vi "digital time using leds.vi"() -> ()   [LabVIEW 2018]
panel:
  out "?":bool
  out "?":bool
  out "?":bool
  out "?":bool
  out "?":bool
  out "?":bool
  out "?":bool
  out "?":bool
  out "?":bool
  out "?":bool
  out "?":bool
  out "?":bool
  out "?":bool
  out "?":bool
  out "?":bool
  out "?":bool
  out "?":bool
  out "?":bool
  out "?":bool
  out "?":bool
  out "?":bool
  out "?":bool
  out "?":bool
  out "?":bool
  out "?":bool
  out "?":bool
  out "?":bool
  out "?":bool
  in  "stop":bool
  out "?":bool
  out "?":bool
  out "?":bool
  out "?":bool
  out "?":bool
  out "?":bool
  out "?":bool
  out "?":bool
  out "?":bool
  out "?":bool
  out "?":bool
  out "?":bool
  out "?":bool
  out "?":bool
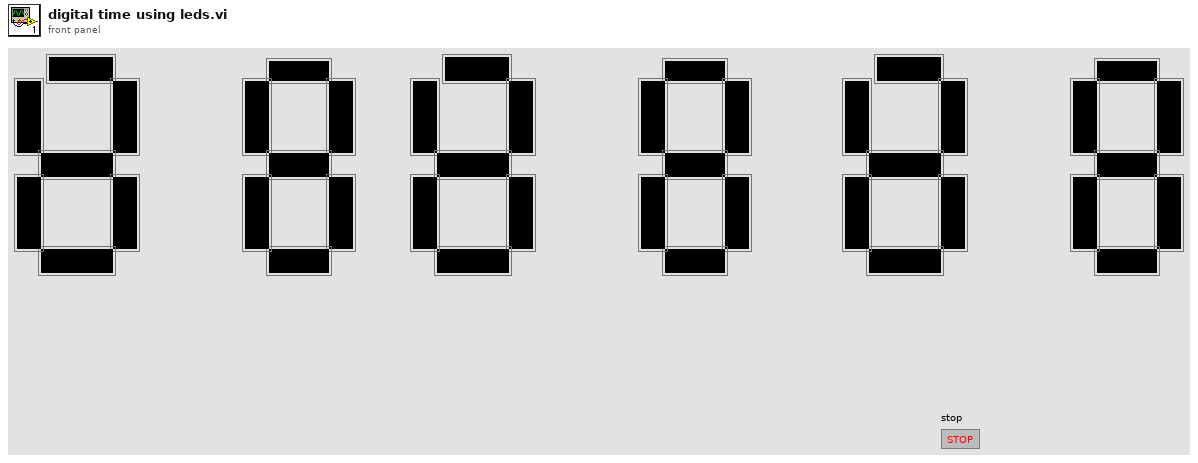
[diagram p1: front panel]
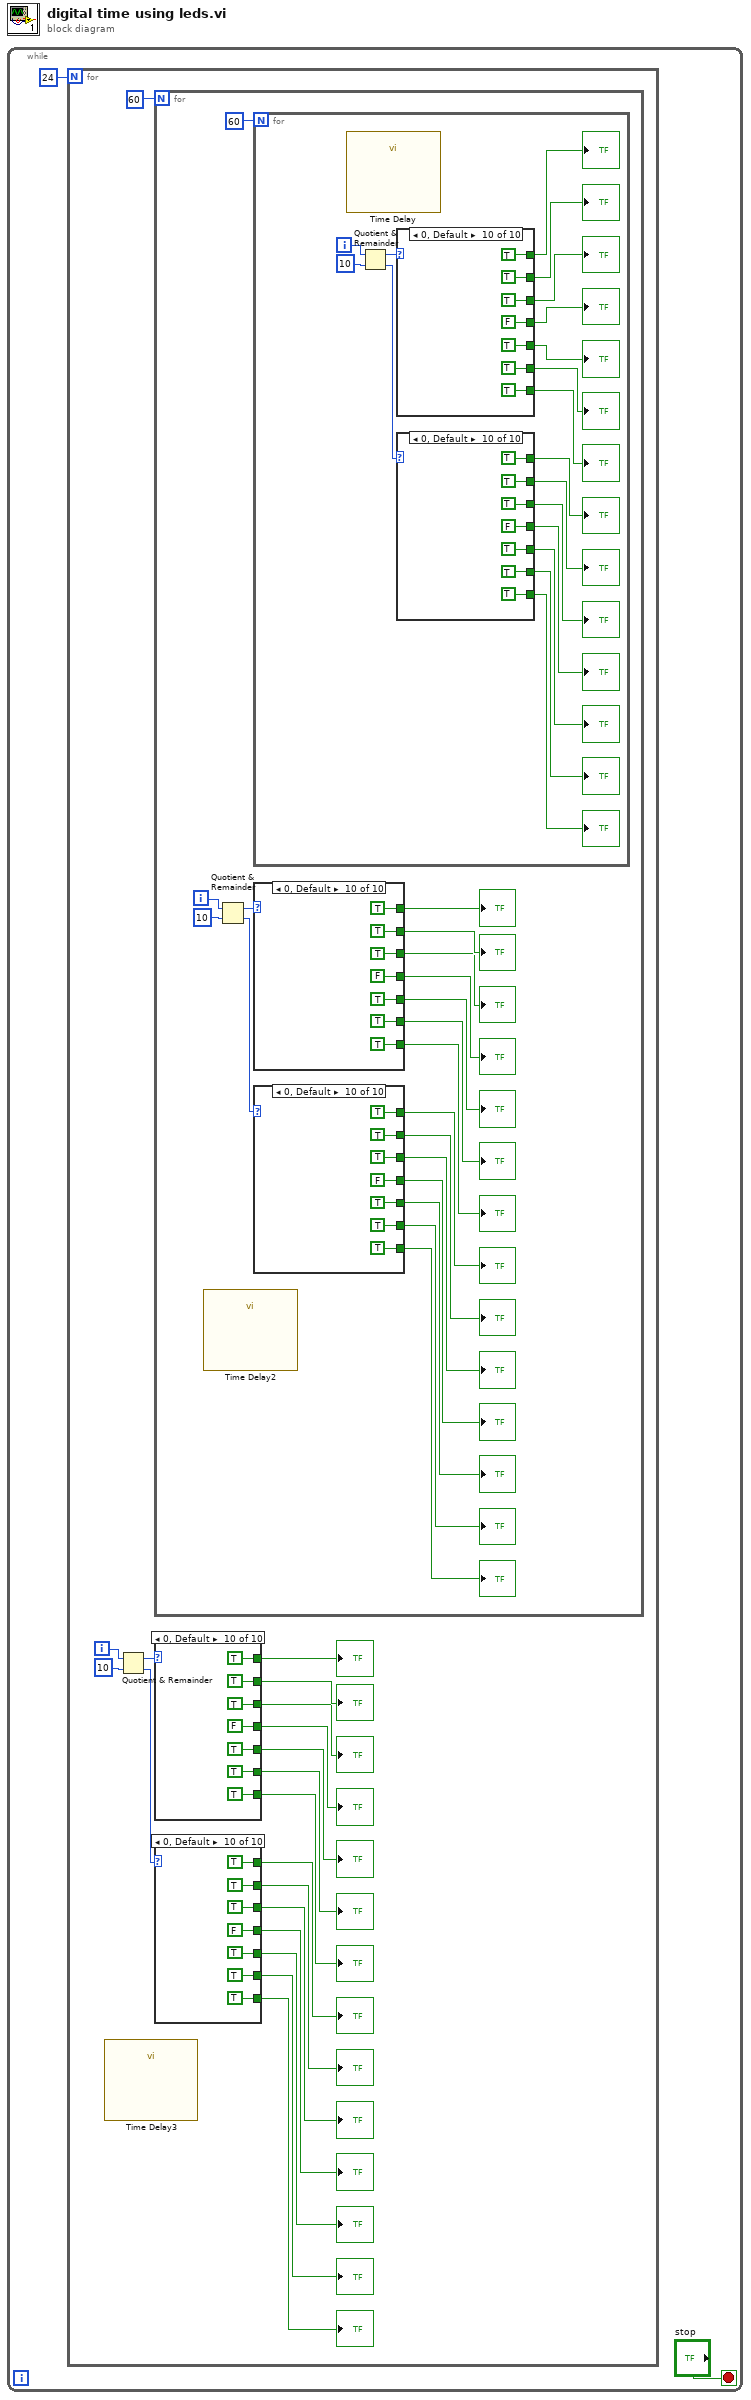
[diagram p0: block diagram]
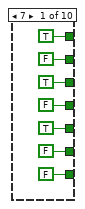
[diagram p2: hidden frame]
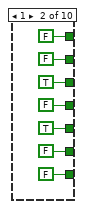
[diagram p3: hidden frame]
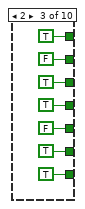
[diagram p4: hidden frame]
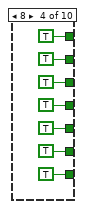
[diagram p5: hidden frame]
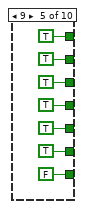
[diagram p6: hidden frame]
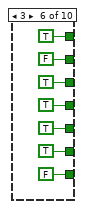
[diagram p7: hidden frame]
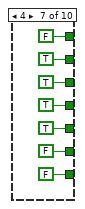
[diagram p8: hidden frame]
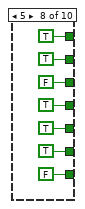
[diagram p9: hidden frame]
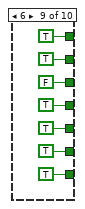
[diagram p10: hidden frame]
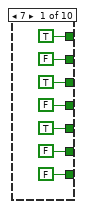
[diagram p11: hidden frame]
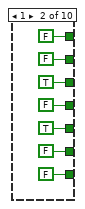
[diagram p12: hidden frame]
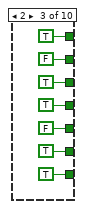
[diagram p13: hidden frame]
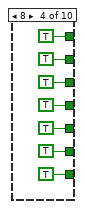
[diagram p14: hidden frame]
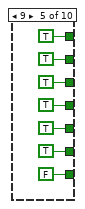
[diagram p15: hidden frame]
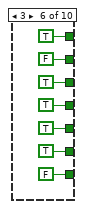
[diagram p16: hidden frame]
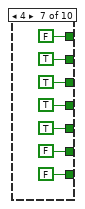
[diagram p17: hidden frame]
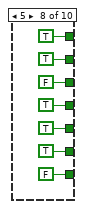
[diagram p18: hidden frame]
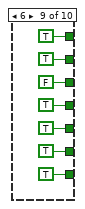
[diagram p19: hidden frame]
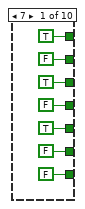
[diagram p20: hidden frame]
diagram:
  n1 = while {
    stop <- "stop" stop-if-true
    n2 = for {
      N: 24 -> [_]
      i -> [w3]
      n3 = call "Time Delay3"() -> ()  [unwired: 11 in, 1 out]
      n4 = Quotient & Remainder(x=w3, y=10) -> (x-y*floor(x/y)=w5:i32, floor(x/y)=w4:i32)
      n5 = for {
        N: 60 -> [_]
        i -> [w163]
        n6 = call "Time Delay2"() -> ()  [unwired: 11 in, 1 out]
        n7 = Quotient & Remainder(x=w163, y=10) -> (x-y*floor(x/y)=w164:i32, floor(x/y)=w162:i32)
        n8 = for {
          N: 60 -> [_]
          i -> [w331]
          n9 = call "Time Delay"() -> ()  [unwired: 11 in, 1 out]
          n10 = Quotient & Remainder(x=w331, y=10) -> (x-y*floor(x/y)=w321:i32, floor(x/y)=w329:i32)
          n11 = case shown="0, Default" w321 {
            tunnel: [TRUE FALSE TRUE TRUE TRUE TRUE FALSE TRUE TRUE TRUE] -> w328
            tunnel: [FALSE FALSE FALSE TRUE TRUE FALSE TRUE TRUE TRUE TRUE] -> w327
            tunnel: [TRUE TRUE TRUE TRUE TRUE TRUE TRUE FALSE FALSE TRUE] -> w326
            tunnel: [FALSE FALSE TRUE TRUE TRUE TRUE TRUE TRUE TRUE FALSE] -> w325
            tunnel: [TRUE TRUE FALSE TRUE TRUE TRUE TRUE TRUE TRUE TRUE] -> w324
            tunnel: [FALSE FALSE TRUE TRUE TRUE TRUE FALSE TRUE TRUE TRUE] -> w323
            tunnel: [FALSE FALSE TRUE TRUE FALSE FALSE FALSE FALSE TRUE TRUE] -> w322
            frame 7 {
            }
            frame 1 {
            }
            frame 2 {
            }
            frame 8 {
            }
            frame 9 {
            }
            frame 3 {
            }
            frame 4 {
            }
            frame 5 {
            }
            frame 6 {
            }
            frame 0, Default {
            }
          }
          "?" <- w328
          "?" <- w327
          "?" <- w326
          "?" <- w325
          "?" <- w324
          "?" <- w323
          "?" <- w322
          n12 = case shown="0, Default" w329 {
            tunnel: [TRUE FALSE TRUE TRUE TRUE TRUE FALSE TRUE TRUE TRUE] -> w338
            tunnel: [FALSE FALSE FALSE TRUE TRUE FALSE TRUE TRUE TRUE TRUE] -> w337
            tunnel: [TRUE TRUE TRUE TRUE TRUE TRUE TRUE FALSE FALSE TRUE] -> w336
            tunnel: [FALSE FALSE TRUE TRUE TRUE TRUE TRUE TRUE TRUE FALSE] -> w335
            tunnel: [TRUE TRUE FALSE TRUE TRUE TRUE TRUE TRUE TRUE TRUE] -> w334
            tunnel: [FALSE FALSE TRUE TRUE TRUE TRUE FALSE TRUE TRUE TRUE] -> w333
            tunnel: [FALSE FALSE TRUE TRUE FALSE FALSE FALSE FALSE TRUE TRUE] -> w332
            frame 7 {
            }
            frame 1 {
            }
            frame 2 {
            }
            frame 8 {
            }
            frame 9 {
            }
            frame 3 {
            }
            frame 4 {
            }
            frame 5 {
            }
            frame 6 {
            }
            frame 0, Default {
            }
          }
          "?" <- w338
          "?" <- w337
          "?" <- w336
          "?" <- w335
          "?" <- w334
          "?" <- w333
          "?" <- w332
        }
        n13 = case shown="0, Default" w164 {
          tunnel: [TRUE FALSE TRUE TRUE TRUE TRUE FALSE TRUE TRUE TRUE] -> w171
          tunnel: [FALSE FALSE FALSE TRUE TRUE FALSE TRUE TRUE TRUE TRUE] -> w170
          tunnel: [TRUE TRUE TRUE TRUE TRUE TRUE TRUE FALSE FALSE TRUE] -> w169
          tunnel: [FALSE FALSE TRUE TRUE TRUE TRUE TRUE TRUE TRUE FALSE] -> w168
          tunnel: [TRUE TRUE FALSE TRUE TRUE TRUE TRUE TRUE TRUE TRUE] -> w167
          tunnel: [FALSE FALSE TRUE TRUE TRUE TRUE FALSE TRUE TRUE TRUE] -> w166
          tunnel: [FALSE FALSE TRUE TRUE FALSE FALSE FALSE FALSE TRUE TRUE] -> w165
          frame 7 {
          }
          frame 1 {
          }
          frame 2 {
          }
          frame 8 {
          }
          frame 9 {
          }
          frame 3 {
          }
          frame 4 {
          }
          frame 5 {
          }
          frame 6 {
          }
          frame 0, Default {
          }
        }
        "?" <- w171
        "?" <- w170
        "?" <- w169
        "?" <- w168
        "?" <- w167
        "?" <- w166
        "?" <- w165
        n14 = case shown="0, Default" w162 {
          tunnel: [TRUE FALSE TRUE TRUE TRUE TRUE FALSE TRUE TRUE TRUE] -> w179
          tunnel: [FALSE FALSE FALSE TRUE TRUE FALSE TRUE TRUE TRUE TRUE] -> w178
          tunnel: [TRUE TRUE TRUE TRUE TRUE TRUE TRUE FALSE FALSE TRUE] -> w177
          tunnel: [FALSE FALSE TRUE TRUE TRUE TRUE TRUE TRUE TRUE FALSE] -> w176
          tunnel: [TRUE TRUE FALSE TRUE TRUE TRUE TRUE TRUE TRUE TRUE] -> w175
          tunnel: [FALSE FALSE TRUE TRUE TRUE TRUE FALSE TRUE TRUE TRUE] -> w174
          tunnel: [FALSE FALSE TRUE TRUE FALSE FALSE FALSE FALSE TRUE TRUE] -> w173
          frame 7 {
          }
          frame 1 {
          }
          frame 2 {
          }
          frame 8 {
          }
          frame 9 {
          }
          frame 3 {
          }
          frame 4 {
          }
          frame 5 {
          }
          frame 6 {
          }
          frame 0, Default {
          }
        }
        "?" <- w179
        "?" <- w178
        "?" <- w177
        "?" <- w176
        "?" <- w175
        "?" <- w174
        "?" <- w173
      }
      n15 = case shown="0, Default" w5 {
        tunnel: [TRUE FALSE TRUE TRUE TRUE TRUE FALSE TRUE TRUE TRUE] -> w12
        tunnel: [FALSE FALSE FALSE TRUE TRUE FALSE TRUE TRUE TRUE TRUE] -> w11
        tunnel: [TRUE TRUE TRUE TRUE TRUE TRUE TRUE FALSE FALSE TRUE] -> w10
        tunnel: [FALSE FALSE TRUE TRUE TRUE TRUE TRUE TRUE TRUE FALSE] -> w9
        tunnel: [TRUE TRUE FALSE TRUE TRUE TRUE TRUE TRUE TRUE TRUE] -> w8
        tunnel: [FALSE FALSE TRUE TRUE TRUE TRUE FALSE TRUE TRUE TRUE] -> w7
        tunnel: [FALSE FALSE TRUE TRUE FALSE FALSE FALSE FALSE TRUE TRUE] -> w6
        frame 7 {
        }
        frame 1 {
        }
        frame 2 {
        }
        frame 8 {
        }
        frame 9 {
        }
        frame 3 {
        }
        frame 4 {
        }
        frame 5 {
        }
        frame 6 {
        }
        frame 0, Default {
        }
      }
      "?" <- w12
      "?" <- w11
      "?" <- w10
      "?" <- w9
      "?" <- w8
      "?" <- w7
      "?" <- w6
      n16 = case shown="0, Default" w4 {
        tunnel: [TRUE FALSE TRUE TRUE TRUE TRUE FALSE TRUE TRUE TRUE] -> w20
        tunnel: [FALSE FALSE FALSE TRUE TRUE FALSE TRUE TRUE TRUE TRUE] -> w19
        tunnel: [TRUE TRUE TRUE TRUE TRUE TRUE TRUE FALSE FALSE TRUE] -> w18
        tunnel: [FALSE FALSE TRUE TRUE TRUE TRUE TRUE TRUE TRUE FALSE] -> w17
        tunnel: [TRUE TRUE FALSE TRUE TRUE TRUE TRUE TRUE TRUE TRUE] -> w16
        tunnel: [FALSE FALSE TRUE TRUE TRUE TRUE FALSE TRUE TRUE TRUE] -> w15
        tunnel: [FALSE FALSE TRUE TRUE FALSE FALSE FALSE FALSE TRUE TRUE] -> w14
        frame 7 {
        }
        frame 1 {
        }
        frame 2 {
        }
        frame 8 {
        }
        frame 9 {
        }
        frame 3 {
        }
        frame 4 {
        }
        frame 5 {
        }
        frame 6 {
        }
        frame 0, Default {
        }
      }
      "?" <- w20
      "?" <- w19
      "?" <- w18
      "?" <- w17
      "?" <- w16
      "?" <- w15
      "?" <- w14
    }
  }
